vi "Save Raw RP Data.vi"(8 "error in (no error)":errorcluster, 10 "Raw data":string, 11 "Red Pitaya Digitizer in":refnum<class "Red Pitaya Digitizer.lvclass">) -> (0 "error out":errorcluster, 1 "Finished":bool, 2 "Current read position":i32, 3 "Red Pitaya Digitizer out":refnum<class "Red Pitaya Digitizer.lvclass">)   [LabVIEW 2018, in "Red Pitaya Digitizer.lvclass"]
uses:
  Red Pitaya Digitizer.lvclass
  C:/github/NHMFL_Core/Libraries/Instruments/Pulse Driver/Pulse Driver.lvclass
  Instruments/Pulse Driver/Pulse Driver.lvclass/Pulse Driver.ctl
  Instruments/Pulse Driver/Read Current read position.vi
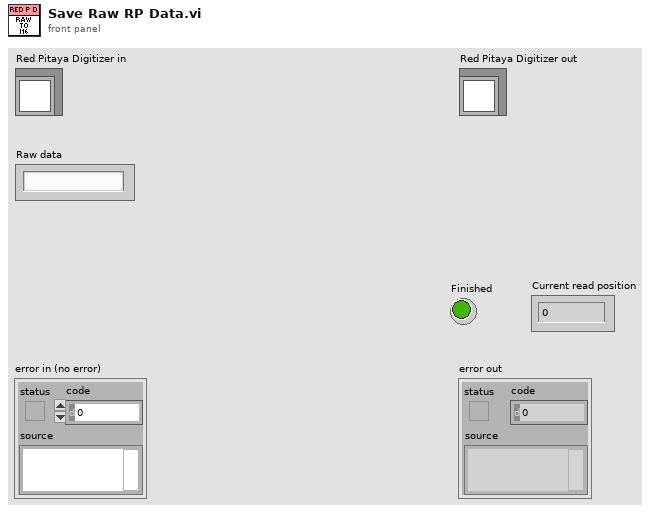
[diagram p1: front panel]
types:
  T1 = enum16{"big-endian, network order", "native, host order", "little-endian"}
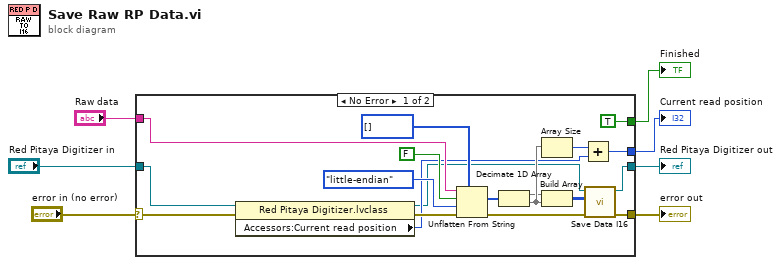
[diagram p0: block diagram]
diagram:
  n1 = case shown="No Error" "error in (no error)" {
    selector: "error in (no error)" -> [w17 w28]
    tunnel: [w9 w28] -> w6
    tunnel: [w11 w27] -> w4
    tunnel: "Red Pitaya Digitizer in" -> [w13 w27]
    tunnel: "Raw data" -> [w19 _]
    tunnel: [w15 _] -> w2
    tunnel: [TRUE ("Finished") _] -> w1
    frame No Error {
      n2 = property class="Red Pitaya Digitizer.lvclass"(reference=w13, error in=w17) -> (reference out=w12:refnum<class "Red Pitaya Digitizer.lvclass">, error out=w18:errorcluster, "Accessors:Current read position"=w16:i32)
      n3 = Unflatten From String(type=i16[] [], binary string=w19, data includes array or string size? (T)=FALSE, byte order (0:big-endian, network order)=T1."little-endian", error in (no error)=w18) -> (value=w21:i16[], error out=w10:errorcluster)  [unwired: 1 out]
      n4 = Decimate 1D Array(w21) -> (w20:i16[], w25:i16[])
      n5 = Array Size(array=w25) -> (size(s)=w26:i32)
      n6 = Build Array(w20, w25) -> (w8:i16[][])
      n7 = Add(x=w26, y=w16) -> (x+y=w15:i32)
      n8 = call-dynamic "Save Data I16.vi"("error in (no error)"=w10, "I16 data"=w8, "Pulse Driver in"=w12) -> ("error out"=w9:errorcluster, "Pulse Driver out"=w11:refnum<class "Red Pitaya Digitizer.lvclass">)  [unwired: 7 in]
    }
    frame Error {
    }
  }
  "error out" <- w6
  "Red Pitaya Digitizer out" <- w4
  "Finished" <- w1
  "Current read position" <- w2
